vi ".INI WRITE.vi"(0 "Enum":enum16{"READ", "WRITE"}(ring), 1 "CH 1":dbl, 2 "CH 2":dbl, 3 "CH 3":dbl, 4 "CH 4":dbl, 5 "CH 5":dbl, 6 "CH 6":dbl, 7 "CH 7":dbl, 9 "CH 8":dbl, 10 "Serial Number":T1="0000310", 11 "CH 9":dbl, 13 "CH 10":dbl, 15 "COM":string, 17 "TOL 7":dbl, 18 "MODE":string(combo) caption="Combo Box", 19 "TOL 10":dbl, 20 "TOL 1":dbl, 21 "TOL 2":dbl, 22 "TOL 3":dbl, 23 "TOL 4":dbl, 24 "TOL 5":dbl, 25 "TOL 6":dbl, 26 "TOL 8":dbl, 27 "TOL 9":dbl) -> ()   [LabVIEW 2021]
uses:
  SERIAL N0.ctl
  <vilib>/Utility/config.llb/Read Key (String).vi
  <vilib>/Utility/config.llb/Write Key (Double).vi
  <vilib>/Utility/config.llb/Write Key (String).vi
  <vilib>/Utility/config.llb/NI_LVConfig.lvlib
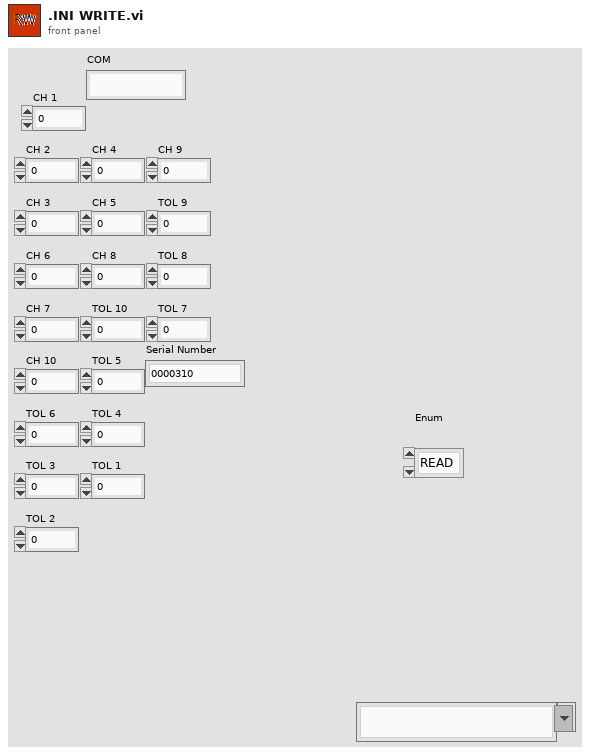
[diagram p1: front panel]
types:
  T1 = typedef "SERIAL N0.ctl" = string
  T2 = typedef "NI_LVConfig.lvlib/Config Data RefNum.ctl" = refnum<k1>
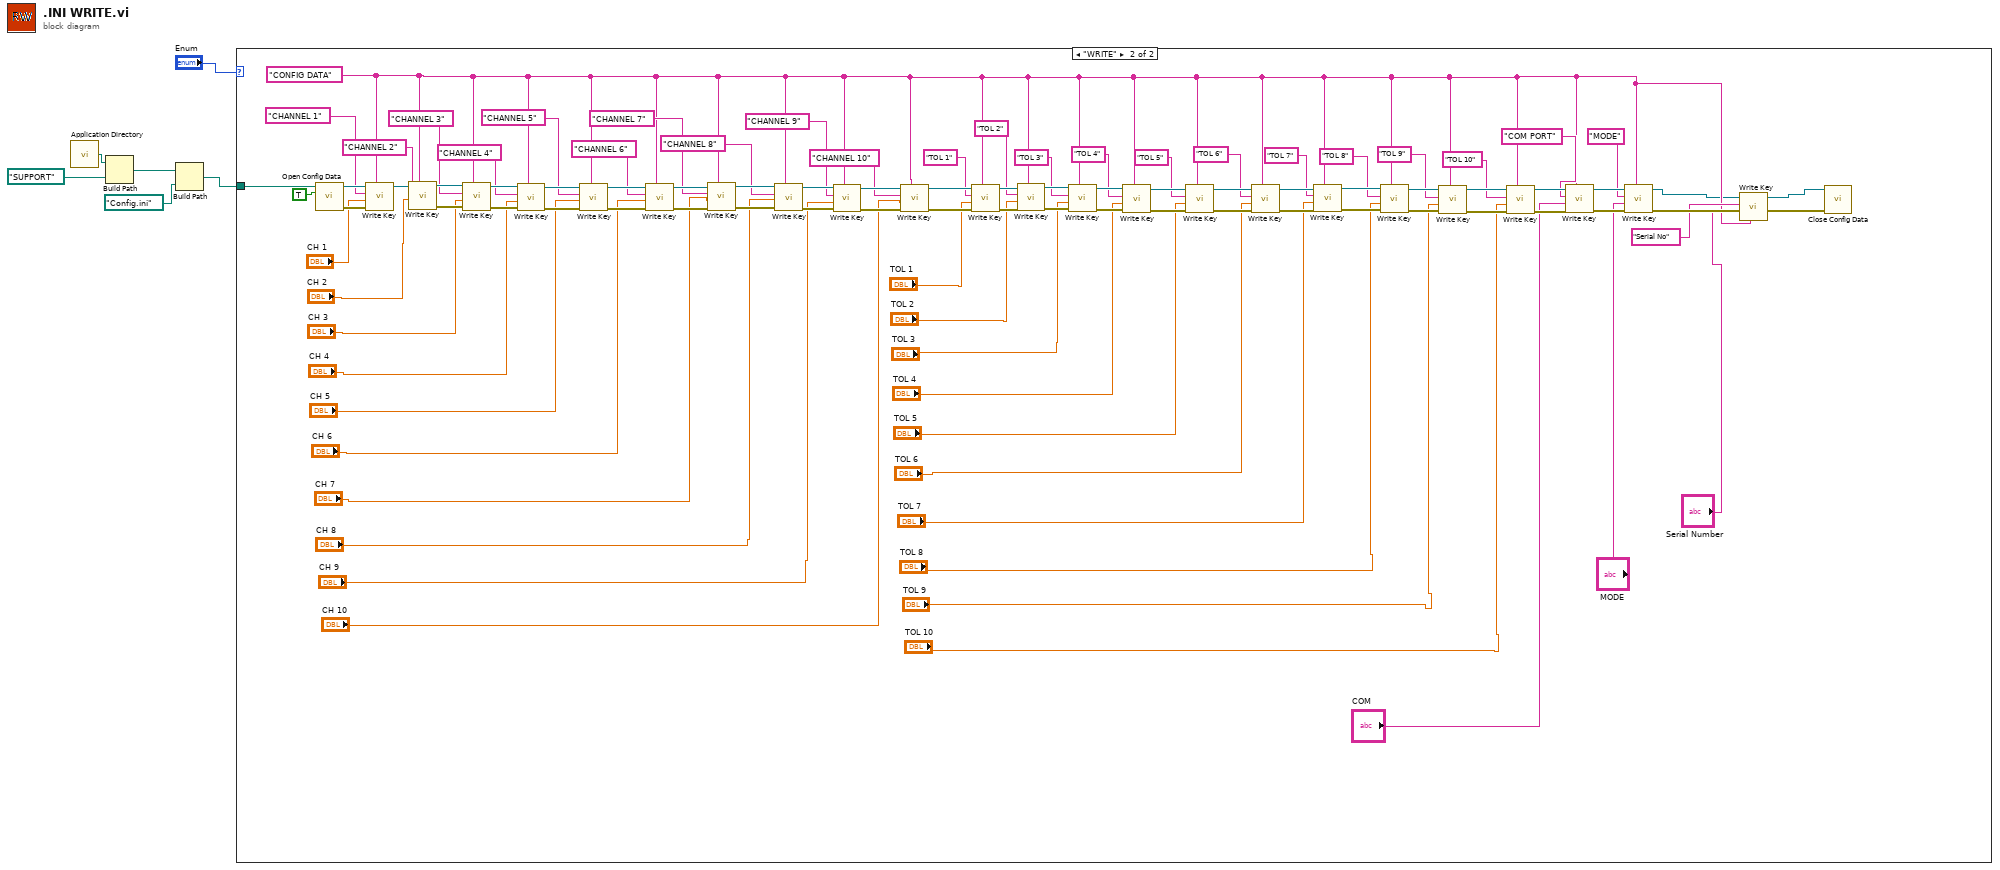
[diagram p0: block diagram]
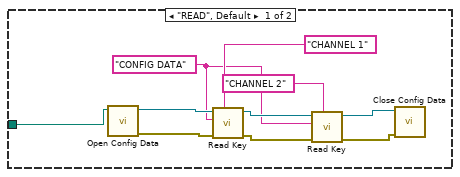
[diagram p2: hidden frame]
diagram:
  n1 = call <vilib>:"Application Directory.vi"() -> ("Application Directory"=w5:path)
  n2 = Build Path(base path=w5, name or relative path=path "SUPPORT") -> (appended path=w6:path)
  n3 = Build Path(base path=w6, name or relative path=path "Config.ini") -> (appended path=w2:path)
  n4 = case shown="\"WRITE\"" "Enum" {
    tunnel: w2 -> [w16 w108]
    frame "READ", Default {
      w8 = "CONFIG DATA" ("key")
      n5 = call <vilib>:"Open Config Data.vi"("configuration file path"=w16) -> ("error out"=w14:errorcluster, "refnum"=w15:T2)  [unwired: 8 in, 1 out]
      n6 = call-poly <vilib>:"Read Key.vi"("section"="CHANNEL 1", "error in (no error)"=w14, "key"=w8, "refnum"=w15) -> ("error out"=w10:errorcluster, "refnum out"=w12:T2)  [unwired: 4 in, 2 out]
      n7 = call-poly <vilib>:"Read Key.vi"("section"="CHANNEL 2", "error in (no error)"=w10, "key"=w8, "refnum"=w12) -> ("error out"=w9:errorcluster, "refnum out"=w11:T2)  [unwired: 4 in, 2 out]
      n8 = call <vilib>:"Close Config Data.vi"("error in (no error)"=w9, "refnum"=w11) -> ()  [unwired: 8 in, 2 out]
    }
    frame "WRITE" {
      w19 = "CONFIG DATA" ("section")
      n9 = call <vilib>:"Open Config Data.vi"("create file if necessary (T)"=TRUE, "configuration file path"=w108) -> ("error out"=w109:errorcluster, "refnum"=w110:T2)  [unwired: 7 in, 1 out]
      n10 = call-poly <vilib>:"Write Key.vi"("section"=w19, "error in (no error)"=w109, "value"="CH 1", "key"="CHANNEL 1", "refnum"=w110) -> ("refnum out"=w107:T2)  [unwired: 4 in, 2 out]
      n11 = call-poly <vilib>:"Write Key.vi"("section"=w19, "value"="CH 2", "key"="CHANNEL 2", "refnum"=w107) -> ("error out"=w104:errorcluster, "refnum out"=w103:T2)  [unwired: 5 in, 1 out]
      n12 = call-poly <vilib>:"Write Key.vi"("section"=w19, "error in (no error)"=w104, "value"="CH 3", "key"="CHANNEL 3", "refnum"=w103) -> ("error out"=w100:errorcluster, "refnum out"=w101:T2)  [unwired: 4 in, 1 out]
      n13 = call-poly <vilib>:"Write Key.vi"("section"=w19, "error in (no error)"=w100, "value"="CH 4", "key"="CHANNEL 4", "refnum"=w101) -> ("error out"=w97:errorcluster, "refnum out"=w98:T2)  [unwired: 4 in, 1 out]
      n14 = call-poly <vilib>:"Write Key.vi"("section"=w19, "error in (no error)"=w97, "value"="CH 5", "key"="CHANNEL 5", "refnum"=w98) -> ("error out"=w94:errorcluster, "refnum out"=w95:T2)  [unwired: 4 in, 1 out]
      n15 = call-poly <vilib>:"Write Key.vi"("section"=w19, "error in (no error)"=w94, "value"="CH 6", "key"="CHANNEL 6", "refnum"=w95) -> ("error out"=w91:errorcluster, "refnum out"=w92:T2)  [unwired: 4 in, 1 out]
      n16 = call-poly <vilib>:"Write Key.vi"("section"=w19, "error in (no error)"=w91, "value"="CH 7", "key"="CHANNEL 7", "refnum"=w92) -> ("error out"=w89:errorcluster, "refnum out"=w90:T2)  [unwired: 4 in, 1 out]
      n17 = call-poly <vilib>:"Write Key.vi"("section"=w19, "error in (no error)"=w89, "value"="CH 8", "key"="CHANNEL 8", "refnum"=w90) -> ("error out"=w85:errorcluster, "refnum out"=w86:T2)  [unwired: 4 in, 1 out]
      n18 = call-poly <vilib>:"Write Key.vi"("section"=w19, "error in (no error)"=w85, "value"="CH 9", "key"="CHANNEL 9", "refnum"=w86) -> ("error out"=w82:errorcluster, "refnum out"=w83:T2)  [unwired: 4 in, 1 out]
      n19 = call-poly <vilib>:"Write Key.vi"("section"=w19, "error in (no error)"=w82, "value"="CH 10", "key"="CHANNEL 10", "refnum"=w83) -> ("error out"=w79:errorcluster, "refnum out"=w80:T2)  [unwired: 4 in, 1 out]
      n20 = call-poly <vilib>:"Write Key.vi"("section"=w19, "error in (no error)"=w79, "value"="TOL 1", "key"="TOL 1", "refnum"=w80) -> ("error out"=w77:errorcluster, "refnum out"=w78:T2)  [unwired: 4 in, 1 out]
      n21 = call-poly <vilib>:"Write Key.vi"("section"=w19, "error in (no error)"=w77, "value"="TOL 2", "key"="TOL 2", "refnum"=w78) -> ("error out"=w75:errorcluster, "refnum out"=w76:T2)  [unwired: 4 in, 1 out]
      n22 = call-poly <vilib>:"Write Key.vi"("section"=w19, "error in (no error)"=w75, "value"="TOL 3", "key"="TOL 3", "refnum"=w76) -> ("error out"=w73:errorcluster, "refnum out"=w74:T2)  [unwired: 4 in, 1 out]
      n23 = call-poly <vilib>:"Write Key.vi"("section"=w19, "error in (no error)"=w73, "value"="TOL 4", "key"="TOL 4", "refnum"=w74) -> ("error out"=w71:errorcluster, "refnum out"=w72:T2)  [unwired: 4 in, 1 out]
      n24 = call-poly <vilib>:"Write Key.vi"("section"=w19, "error in (no error)"=w71, "value"="TOL 5", "key"="TOL 5", "refnum"=w72) -> ("error out"=w69:errorcluster, "refnum out"=w70:T2)  [unwired: 4 in, 1 out]
      n25 = call-poly <vilib>:"Write Key.vi"("section"=w19, "error in (no error)"=w69, "value"="TOL 6", "key"="TOL 6", "refnum"=w70) -> ("error out"=w67:errorcluster, "refnum out"=w68:T2)  [unwired: 4 in, 1 out]
      n26 = call-poly <vilib>:"Write Key.vi"("section"=w19, "error in (no error)"=w67, "value"="TOL 7", "key"="TOL 7", "refnum"=w68) -> ("error out"=w65:errorcluster, "refnum out"=w66:T2)  [unwired: 4 in, 1 out]
      n27 = call-poly <vilib>:"Write Key.vi"("section"=w19, "error in (no error)"=w65, "value"="TOL 8", "key"="TOL 8", "refnum"=w66) -> ("error out"=w63:errorcluster, "refnum out"=w64:T2)  [unwired: 4 in, 1 out]
      n28 = call-poly <vilib>:"Write Key.vi"("section"=w19, "error in (no error)"=w63, "value"="TOL 9", "key"="TOL 9", "refnum"=w64) -> ("error out"=w61:errorcluster, "refnum out"=w62:T2)  [unwired: 4 in, 1 out]
      n29 = call-poly <vilib>:"Write Key.vi"("section"=w19, "error in (no error)"=w61, "value"="TOL 10", "key"="TOL 10", "refnum"=w62) -> ("error out"=w29:errorcluster, "refnum out"=w30:T2)  [unwired: 4 in, 1 out]
      n30 = call-poly <vilib>:"Write Key.vi"("section"=w19, "error in (no error)"=w29, "value"="COM", "key"="COM PORT", "refnum"=w30) -> ("error out"=w26:errorcluster, "refnum out"=w27:T2)  [unwired: 4 in, 1 out]
      n31 = call-poly <vilib>:"Write Key.vi"("section"=w19, "error in (no error)"=w26, "value"="MODE", "key"="MODE", "refnum"=w27) -> ("error out"=w22:errorcluster, "refnum out"=w18:T2)  [unwired: 4 in, 1 out]
      n32 = call-poly <vilib>:"Write Key.vi"("section"=w19, "value"="Serial Number", "key"="Serial No", "refnum"=w18) -> ("refnum out"=w17:T2)  [unwired: 5 in, 2 out]
      n33 = call <vilib>:"Close Config Data.vi"("error in (no error)"=w22, "refnum"=w17) -> ()  [unwired: 8 in, 2 out]
    }
  }
